vi "Convert String Array to INI Value.vi"(11 "String Array":string[](array[string])) -> (3 "INI Value":string)   [LabVIEW 2020, in "VI Properties Editor.lvlib"]
doc: "Converts <B>String Array</B> to a corresponding INI key value."
uses:
  VI Properties Editor.lvlib
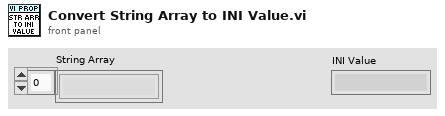
[diagram p1: front panel]
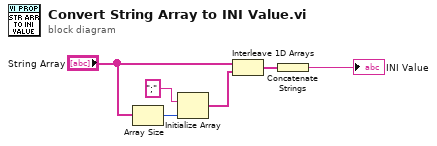
[diagram p0: block diagram]
diagram:
  n1 = Array Size(array="String Array") -> (size(s)=w6:i32)
  n2 = Initialize Array(";" ("Separator (,)"), w6) -> (w5:string[])
  n3 = Interleave 1D Arrays("String Array", w5) -> (w4:string[])
  n4 = Concatenate Strings(w4) -> (→"INI Value":string)
